vi "Get WLAN Type.vi"(8 "error in (no error)":errorcluster, 11 "niDTS WLAN Dut Data in":refnum<class "niDTS WLAN Dut Data.lvclass">) -> (0 "error out":errorcluster, 2 "WLAN Type":cluster{"Value":T1, "Init":bool}={"Value"=enum."n - MCS7", "Init"=FALSE}, 3 "niDTS WLAN Dut Data out":refnum<class "niDTS WLAN Dut Data.lvclass">)   [LabVIEW 2015, in "niDTS WLAN.lvlib" / "niDTS WLAN Dut Data.lvclass"]
uses:
  niDTS WLAN Dut Data.lvclass
  Includes/niDTS WLAN INC Type.ctl
  niDTS WLAN Dut Data.lvclass/niDTS WLAN Dut Data.ctl
  niDTS WLAN.lvlib
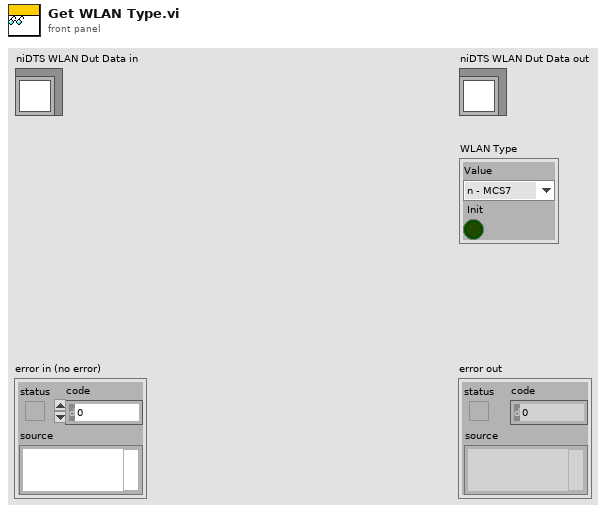
[diagram p1: front panel]
types:
  T1 = typedef "niDTS WLAN.lvlib/niDTS WLAN INC Type.ctl" = enum16{"b - 1 Mbps", "b - 2 Mbps", "b - 5.5 Mbps", "b - 11 Mbps", "ag - 6 Mbps", "ag - 9 Mbps", "ag - 12 Mbps", "ag - 18 Mbps", "ag - 24 Mbps", "ag - 36 Mbps", "ag - 48 Mbps", "ag - 54 Mbps", "n - MCS0", "n - MCS1", "n - MCS2", "n - MCS3", "n - MCS4", "n - MCS5", "n - MCS6", "n - MCS7", "n - MCS8", "n - MCS9", "n - MCS10", "n - MCS11", "n - MCS12", "n - MCS13", "n - MCS14", "n - MCS15", "n - MCS16", "n - MCS17", "n - MCS18", "n - MCS19", "n - MCS20", "n - MCS21", "n - MCS22", "n - MCS23", "n - MCS24", "n - MCS25", "n - MCS26", "n - MCS27", "n - MCS28", "n - MCS29", "n - MCS30", "n - MCS31", "ac - MCS0 -1", "ac - MCS1 -1", "ac - MCS2 -1", "ac - MCS3 -1", "ac - MCS4 -1", "ac - MCS5 -1", "ac - MCS6 -1", "ac - MCS7 -1", "ac - MCS8 -1", "ac - MCS9 -1", "ac - MCS0 -2", "ac - MCS1 -2", "ac - MCS2 -2", "ac - MCS3 -2", "ac - MCS4 -2", "ac - MCS5 -2", "ac - MCS6 -2", "ac - MCS7 -2", "ac - MCS8 -2", "ac - MCS9 -2", "ac - MCS0 -3", "ac - MCS1 -3", "ac - MCS2 -3", "ac - MCS3 -3", "ac - MCS4 -3", "ac - MCS5 -3", "ac - MCS6 -3", "ac - MCS7 -3", "ac - MCS8 -3", "ac - MCS9 -3", "ac - MCS0 -4", "ac - MCS1 -4", "ac - MCS2 -4", "ac - MCS3 -4", "ac - MCS4 -4", "ac - MCS5 -4", "ac - MCS6 -4", "ac - MCS7 -4", "ac - MCS8 -4", "ac - MCS9 -4"}
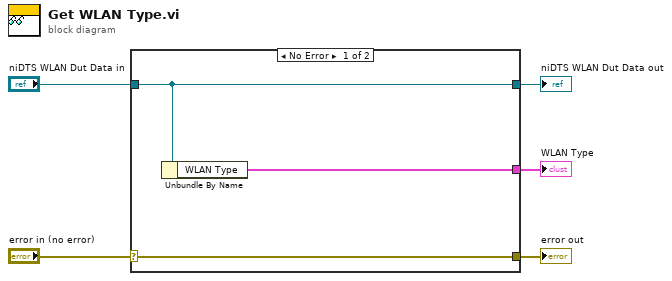
[diagram p0: block diagram]
diagram:
  n1 = case shown="No Error" "error in (no error)" {
    selector: "error in (no error)" -> [w8 w9]
    tunnel: [w8 w9] -> w4
    tunnel: [w7 w10] -> w2
    tunnel: "niDTS WLAN Dut Data in" -> [w7 w10]
    tunnel: [w6 _] -> w1
    frame No Error {
      n2 = Unbundle By Name(w7) -> ("WLAN Type"=w6:cluster{"Value":T1, "Init":bool})
    }
    frame Error {
    }
  }
  "error out" <- w4
  "niDTS WLAN Dut Data out" <- w2
  "WLAN Type" <- w1
